vi "NoodleGrabberSpikeToggle.vi"   [LabVIEW 2014]
uses:
  <vilib>/Rock Robotics/WPI/Relay/WPI_RelayValue.ctl
  Global Variables.vi
types:
  T1 = typedef "WPI_RelayValue.ctl" = enum16{"Off", "On", "Forward", "Reverse"}
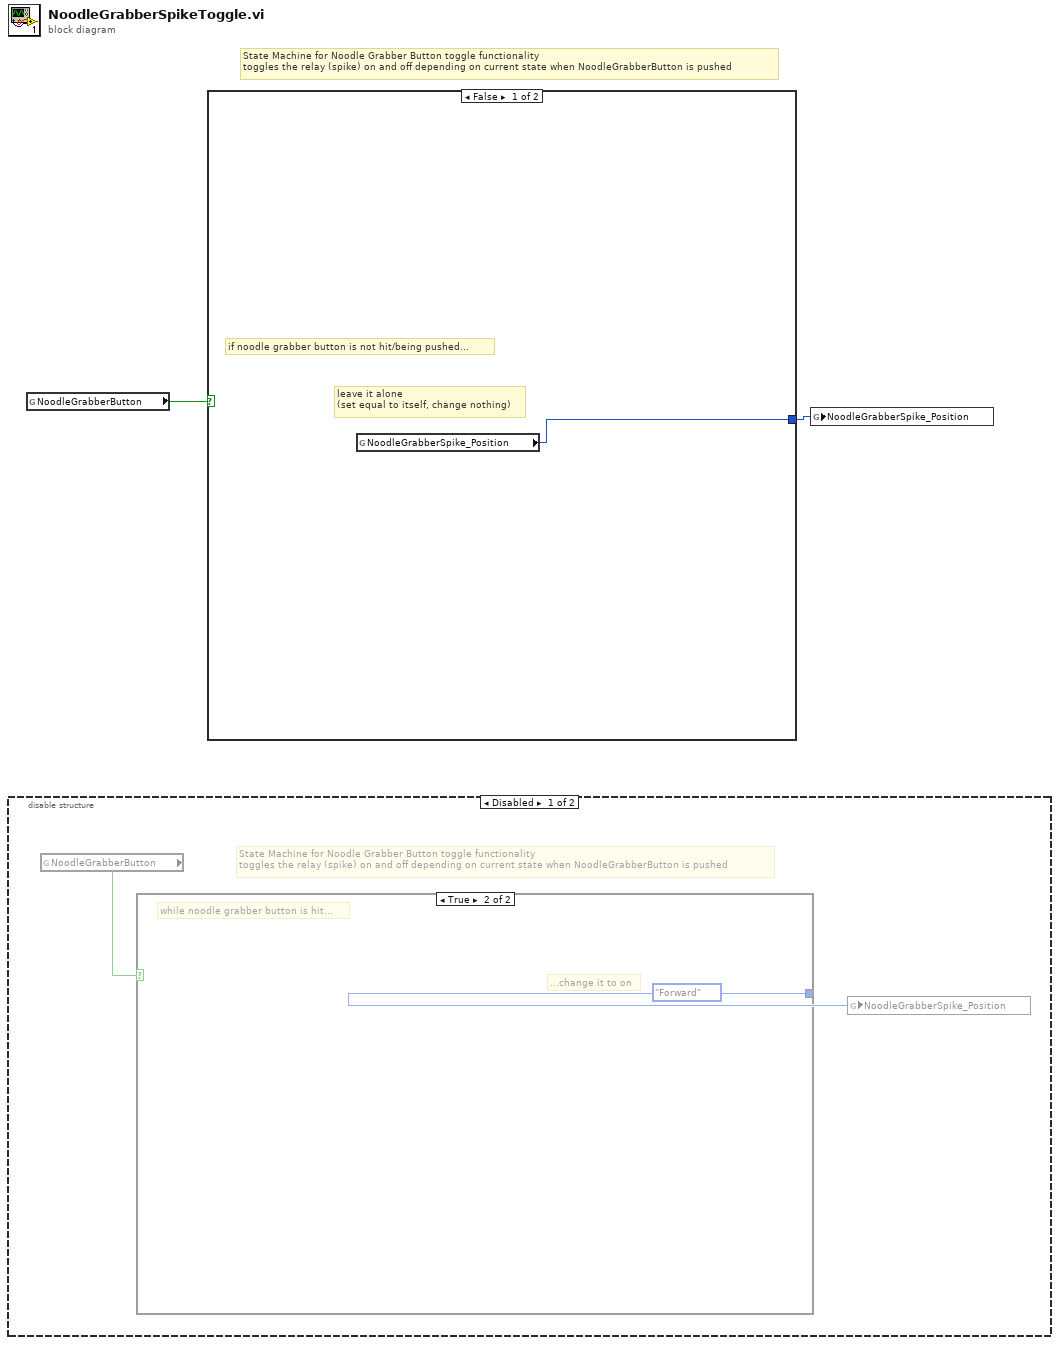
[diagram p0: block diagram]
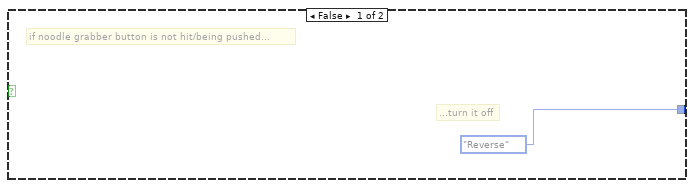
[diagram p2: hidden frame]
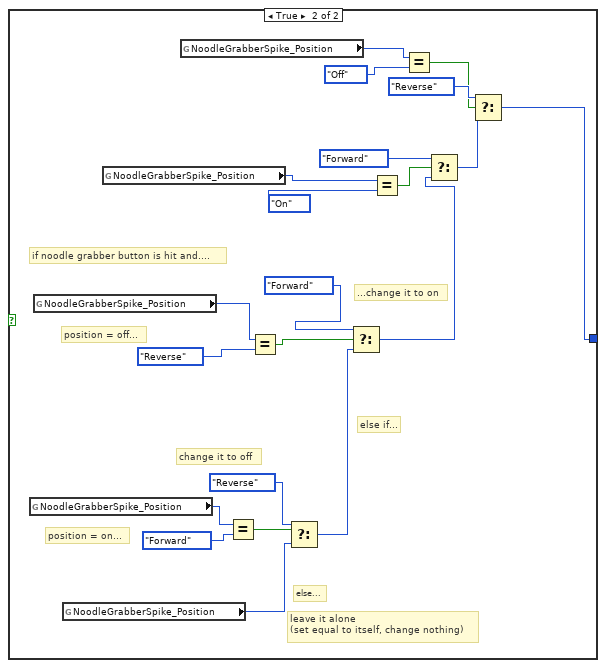
[diagram p4: hidden frame]
diagram:
  # "State Machine for Noodle Grabber Button toggle functionality\ntoggles the relay (spike) on and off depending on current state when NoodleGrabberButton is pushed"
  n1 = disable-structure shown="Disabled" {
    frame Disabled {
      # "State Machine for Noodle Grabber Button toggle functionality\ntoggles the relay (spike) on and off depending on current state when NoodleGrabberButton is pushed"
      n2 = global read "Global Variables.vi" "NoodleGrabberButton"() -> (w3:bool)
      n3 = case shown="True" w3 {
        tunnel: [WPI_RelayValue."Reverse" ("RelayValue") WPI_RelayValue."Forward" ("RelayValue")] -> w4
        frame False {
          # "...turn it off"
          # "if noodle grabber button is not hit/being pushed..."
        }
        frame True {
          # "...change it to on"
          # "while noodle grabber button is hit..."
        }
      }
      n4 = global write "Global Variables.vi" "NoodleGrabberSpike_Position"(w4) -> ()
    }
    frame Enabled {
    }
  }
  n5 = global read "Global Variables.vi" "NoodleGrabberButton"() -> (w2:bool)
  n6 = case shown="False" w2 {
    tunnel: [w7 w8] -> w1
    frame False {
      # "leave it alone\n(set equal to itself, change nothing)"
      # "if noodle grabber button is not hit/being pushed..."
      n7 = global read "Global Variables.vi" "NoodleGrabberSpike_Position"() -> (w7:T1)
    }
    frame True {
      # "else..."
      # "change it to off"
      # "leave it alone\n(set equal to itself, change nothing)"
      # "position = on..."
      # "else if..."
      # "...change it to on"
      # "position = off..."
      # "if noodle grabber button is hit and...."
      n8 = global read "Global Variables.vi" "NoodleGrabberSpike_Position"() -> (w24:T1)
      n9 = global read "Global Variables.vi" "NoodleGrabberSpike_Position"() -> (w25:T1)
      n10 = global read "Global Variables.vi" "NoodleGrabberSpike_Position"() -> (w19:T1)
      n11 = global read "Global Variables.vi" "NoodleGrabberSpike_Position"() -> (w16:T1)
      n12 = global read "Global Variables.vi" "NoodleGrabberSpike_Position"() -> (w11:T1)
      n13 = Equal?(x=w24, y=WPI_RelayValue."Forward" ("RelayValue")) -> (x = y?=w22:bool)
      n14 = Equal?(x=w25, y=WPI_RelayValue."Reverse" ("RelayValue")) -> (x = y?=w27:bool)
      n15 = Select(t=WPI_RelayValue."Reverse" ("RelayValue"), s=w22, f=w19) -> (s? t:f=w21:T1)
      n16 = Select(t=WPI_RelayValue."Forward" ("RelayValue"), s=w27, f=w21) -> (s? t:f=w9:T1)
      n17 = Equal?(x=w16, y=WPI_RelayValue."On" ("NoodleGrabberSpike_Position")) -> (x = y?=w15:bool)
      n18 = Equal?(x=w11, y=WPI_RelayValue."Off" ("NoodleGrabberSpike_Position")) -> (x = y?=w12:bool)
      n19 = Select(t=WPI_RelayValue."Forward" ("NoodleGrabberSpike_Position"), s=w15, f=w9) -> (s? t:f=w18:T1)
      n20 = Select(t=WPI_RelayValue."Reverse" ("NoodleGrabberSpike_Position"), s=w12, f=w18) -> (s? t:f=w8:T1)
    }
  }
  n21 = global write "Global Variables.vi" "NoodleGrabberSpike_Position"(w1) -> ()
